vi "Thermometer.vi"() -> ()   [LabVIEW 2019]
panel:
  out "Temp 2":dbl(slide) scale=0.0..100.0
  out "TempIn":string
  in  "F?":bool
  out "Temp":dbl(slide) scale=0.0..100.0
  in  "Temp":dbl
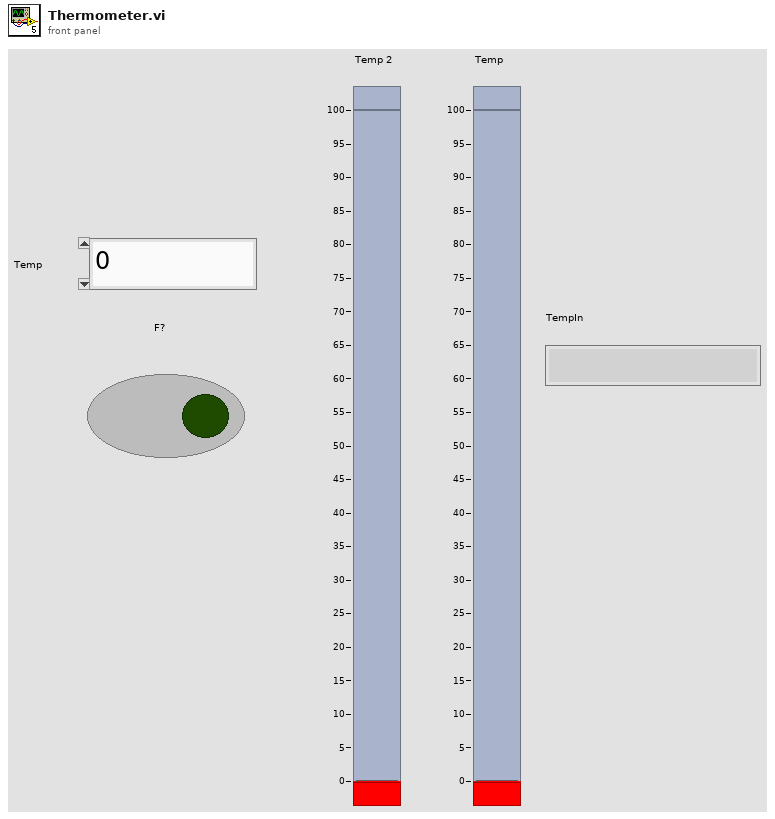
[diagram p1: front panel]
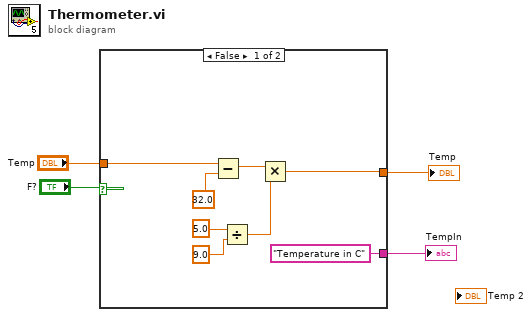
[diagram p0: block diagram]
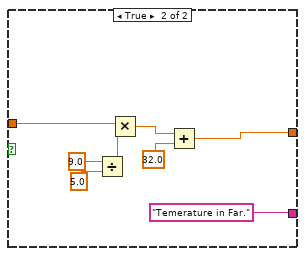
[diagram p2: hidden frame]
diagram:
  n1 = case shown="False" "F?" {
    tunnel: "Temp" -> [w12 w20]
    tunnel: [w6 w14] -> w2
    tunnel: ["Temperature in C" "Temerature in Far."] -> w1
    frame False {
      n2 = Subtract(x=w12, y=32.0) -> (x-y=w10:dbl)
      n3 = Divide(x=5.0, y=9.0) -> (x/y=w7:dbl)
      n4 = Multiply(x=w10, y=w7) -> (x*y=w6:dbl)
    }
    frame True {
      n5 = Divide(x=9.0, y=5.0 ("x")) -> (x/y=w17:dbl)
      n6 = Multiply(x=w20, y=w17) -> (x*y=w16:dbl)
      n7 = Add(x=w16, y=32.0 ("x")) -> (x+y=w14:dbl)
    }
  }
  "Temp" <- w2
  "TempIn" <- w1
